vi "Allowed Variables from string.vi"(5 "config array 2":string[][](array[string])) -> (1 "appended array":string[][](array[string]))   [LabVIEW 2009]
panel:
  out "index of element":i32
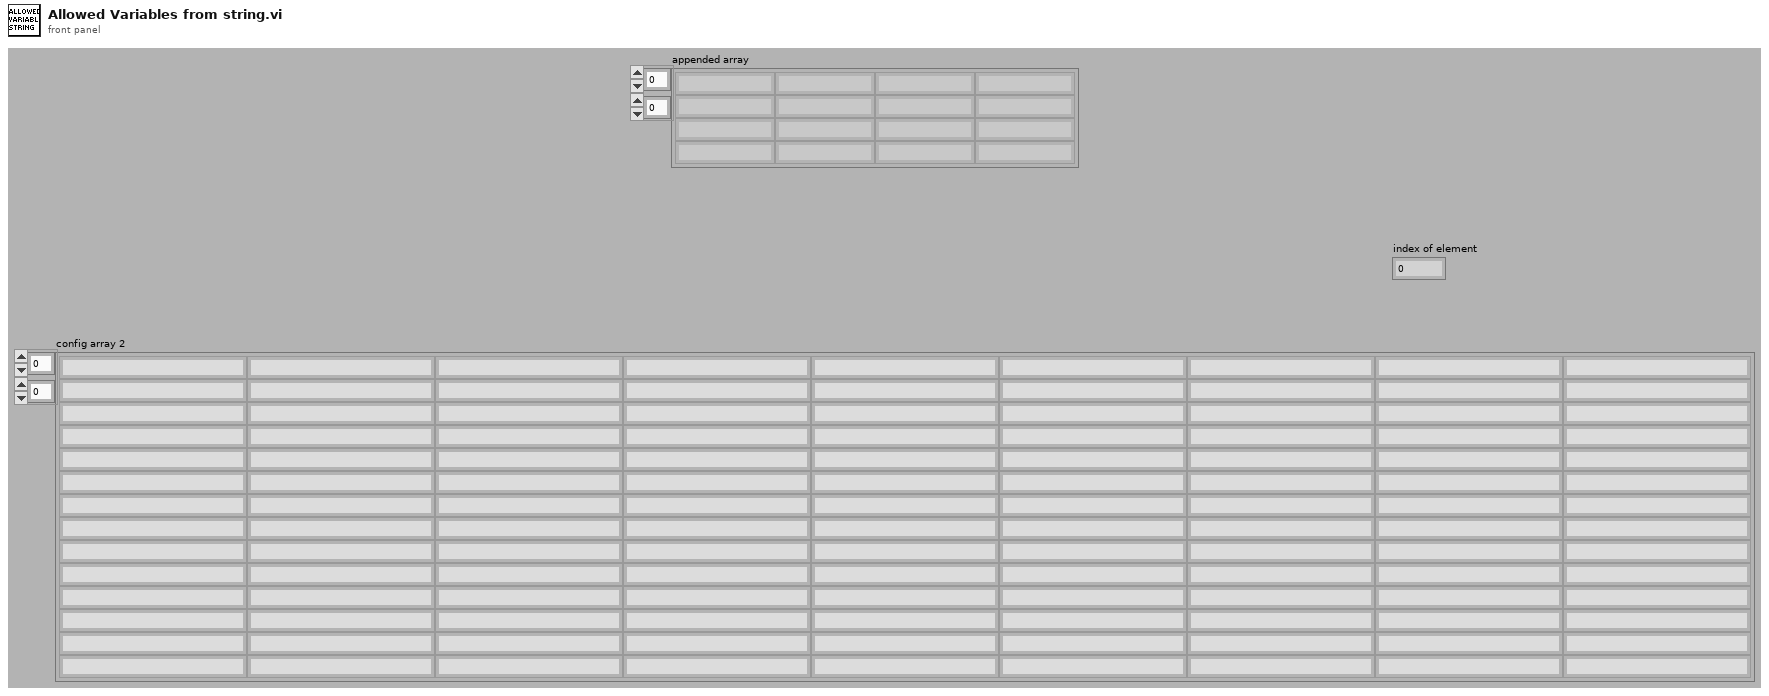
[diagram p1: front panel]
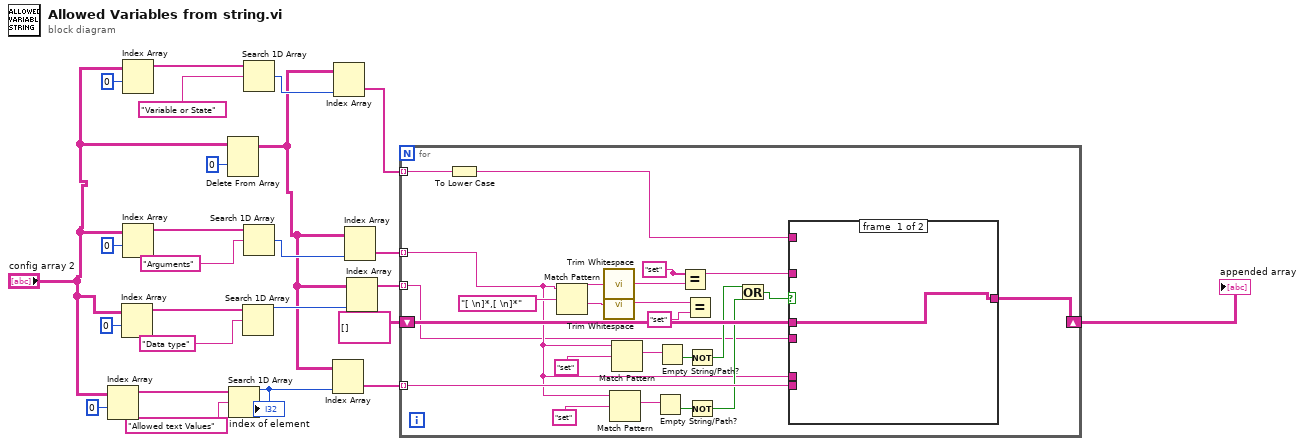
[diagram p0: block diagram]
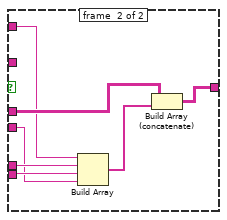
[diagram p2: hidden frame]
diagram:
  n1 = Index Array(array="config array 2", index (row)=0) -> (element=w7:string[])  [unwired: 1 in]
  n2 = Index Array(array="config array 2", index (row)=0) -> (element=w12:string[])  [unwired: 1 in]
  n3 = Index Array(array="config array 2", index (row)=0) -> (element=w20:string[])  [unwired: 1 in]
  n4 = Index Array(array="config array 2", index (row)=0) -> (element=w24:string[])  [unwired: 1 in]
  n5 = Delete From Array(array="config array 2", index (row)=0) -> (array with subset deleted=w4:string[][])  [unwired: 2 in, 1 out]
  n6 = Search 1D Array(1D array=w7, element="Allowed text Values") -> (index of element=w9:i32)  [unwired: 1 in]
  "index of element" <- w9
  n7 = Search 1D Array(1D array=w12, element="Data type") -> (index of element=w10:i32)  [unwired: 1 in]
  n8 = Search 1D Array(1D array=w20, element="Variable or State") -> (index of element=w19:i32)  [unwired: 1 in]
  n9 = Search 1D Array(1D array=w24, element="Arguments") -> (index of element=w23:i32)  [unwired: 1 in]
  n10 = Index Array(array=w4, index (col)=w9) -> (element=w3:string[])  [unwired: 1 in]
  n11 = Index Array(array=w4, index (col)=w19) -> (element=w18:string[])  [unwired: 1 in]
  n12 = Index Array(array=w4, index (col)=w23) -> (element=w15:string[])  [unwired: 1 in]
  n13 = Index Array(array=w4, index (col)=w10) -> (element=w1:string[])  [unwired: 1 in]
  n14 = for {
    shift-right: [w37] -> w2
    shift-left: string[][] [] -> [w38]
    tunnel: w18 -> [w48] mode=indexing
    tunnel: w15 -> [w27] mode=indexing
    tunnel: w3 -> [w36] mode=indexing
    tunnel: w1 -> [w26] mode=indexing
    w39 = "set" ("regular expression")
    n15 = To Lower Case(string=w48) -> (all lower case string=w40:string)
    n16 = Match Pattern(string=w27, regular expression="[ \n]*,[ \n]*") -> (before substring=w42:string, after substring=w45:string)  [unwired: 1 in, 2 out]
    n17 = call <vilib>:"Trim Whitespace.vi"("string"=w42) -> ("trimmed string"=w46:string)  [unwired: 1 in]
    n18 = call <vilib>:"Trim Whitespace.vi"("string"=w45) -> ("trimmed string"=w44:string)  [unwired: 1 in]
    n19 = Match Pattern(string=w27, regular expression="set") -> (match substring=w33:string)  [unwired: 1 in, 3 out]
    n20 = Match Pattern(string=w27, regular expression="set") -> (match substring=w34:string)  [unwired: 1 in, 3 out]
    n21 = Empty String/Path?(string/path=w33) -> (empty?=w30:bool)
    n22 = Empty String/Path?(string/path=w34) -> (empty?=w31:bool)
    n23 = Equal?(x=w39, y=w46) -> ()  [unwired: 1 out]
    n24 = Equal?(x=w44, y="set" ("regular expression")) -> ()  [unwired: 1 out]
    n25 = Not(x=w31) -> (.not. x?=w29:bool)
    n26 = Not(x=w30) -> (.not. x?=w28:bool)
    n27 = Or(x=w29, y=w28) -> (x .or. y?=w41:bool)
    n28 = case shown="True" w41 {
      tunnel: w40 -> [_ w54]
      tunnel: w39 -> [_ _]
      tunnel: w38 -> [w49 w56]
      tunnel: [w49 w55] -> w37
      tunnel: w36 -> [_ w52]
      tunnel: w27 -> [_ w53]
      tunnel: w26 -> [_ w50]
      frame #0 {
      }
      frame #1 {
        n29 = Build Array(w54, w53, w52, w50) -> (w51:string[])
        n30 = Build Array (concatenate)(w56, w51) -> (w55:string[][])
      }
    }
  }
  "appended array" <- w2
